vi "AWS-S3-UploadPage.vi"(0 "Mini AWS S3 API":refnum<class "AWS-S3-MiniAPI.lvclass">, 5 "Object Key":string, 7 "Object Bucket":string, 9 "Object Data":string, 11 "error in":errorcluster) -> (4 "Mini AWS S3 API out":refnum<class "AWS-S3-MiniAPI.lvclass">, 6 "ResponseXml":string, 8 "Download Page URL":string, 15 "error out":errorcluster)   [LabVIEW 2012, in "AWS-S3-MiniAPI.lvclass"]
uses:
  AWS-S3-MiniAPI.lvclass
  C:/Users/Administrator/Documents/Deployment-Automation-and-Release-Engineering-in-LabVIEW/Deployment/AWS-SDK/AWSSDK.dll
  AWS-SDK/AWSSDK.dll
  AWS-S3-MiniAPI.lvclass/AWS-S3-MiniAPI.ctl
panel:
  # "Inputs"
  # "Outputs"
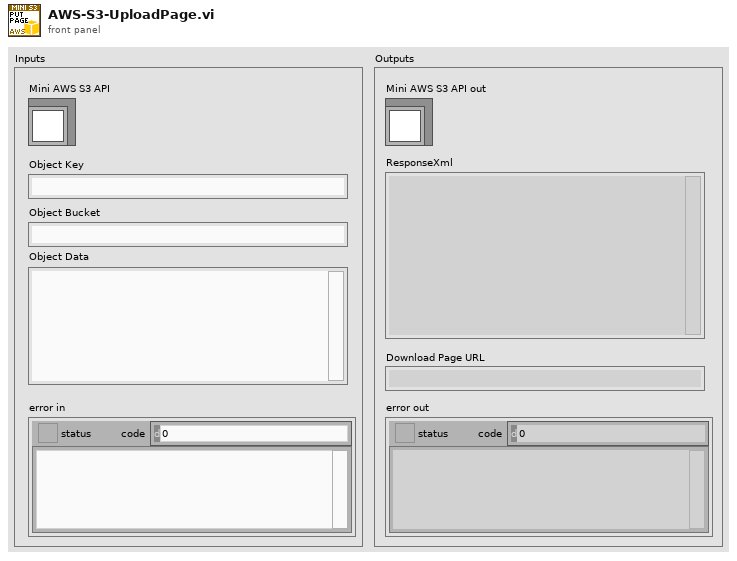
[diagram p1: front panel]
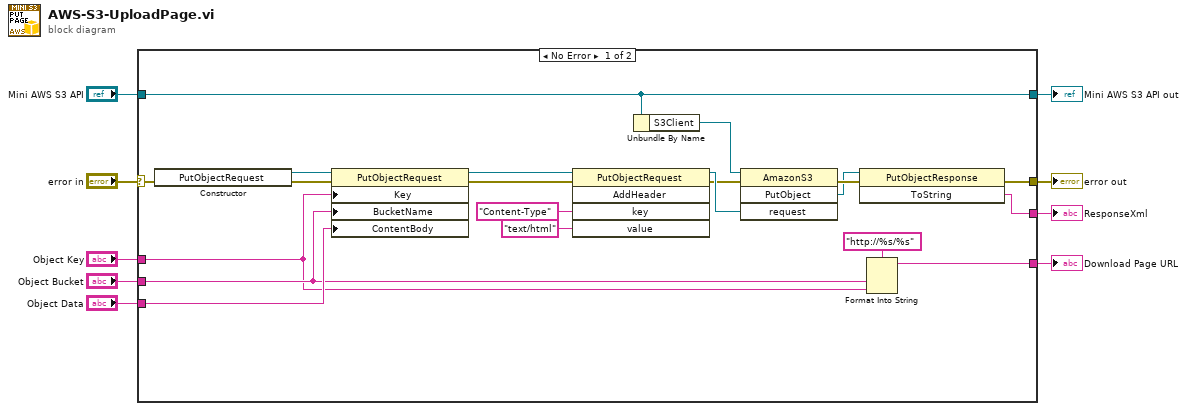
[diagram p0: block diagram]
diagram:
  n1 = case shown="No Error" "error in" {
    selector: "error in" -> [w29 w31]
    tunnel: [w23 w31] -> w9
    tunnel: [w27 w30] -> w7
    tunnel: "Mini AWS S3 API" -> [w27 w30]
    tunnel: "Object Data" -> [w19 _]
    tunnel: "Object Key" -> [w10 _]
    tunnel: "Object Bucket" -> [w12 _]
    tunnel: [w22 _] -> w2
    tunnel: [w11 _] -> w1
    frame No Error {
      n2 = constructor class="PutObjectRequest"(error in=w29) -> (reference out=w26:refnum<k24>, error out=w28:errorcluster)  [unwired: 2 in, 1 out]
      n3 = property class="PutObjectRequest"(reference=w26, error in=w28, "Key"=w10, "BucketName"=w12, "ContentBody"=w19) -> (reference out=w16:refnum<k24>, error out=w15:errorcluster)
      n4 = invoke class="PutObjectRequest" method="AddHeader"(reference=w16, error in=w15, "key"="Content-Type" ("Key"), "value"="text/html" ("Value")) -> (reference out=w20:refnum<k24>, error out=w14:errorcluster)  [unwired: 1 in, 3 out]
      n5 = Unbundle By Name(w27) -> ("S3Client"=w25:refnum<k24>)
      n6 = invoke class="AmazonS3" method="PutObject"(reference=w25, error in=w14, "request"=w20) -> (error out=w24:errorcluster, "PutObject"=w21:refnum<k24>)  [unwired: 1 in, 2 out]
      n7 = invoke class="PutObjectResponse" method="ToString"(reference=w21, error in=w24) -> (error out=w23:errorcluster, "ToString"=w22:string)  [unwired: 1 in, 1 out]
      n8 = Format Into String(format string="http://%s/%s", w12, w10) -> (resulting string=w11:string)  [unwired: 2 in, 1 out]
    }
    frame Error {
    }
  }
  "error out" <- w9
  "Mini AWS S3 API out" <- w7
  "ResponseXml" <- w2
  "Download Page URL" <- w1
